vi "Read Username.vi"(8 "error in (no error)":errorcluster, 11 "Player in":refnum<class "Player.lvclass">) -> (0 "error out":errorcluster, 2 "Username":string, 3 "Player out":refnum<class "Player.lvclass">)   [LabVIEW 2019, in "Player.lvclass"]
uses:
  Player.lvclass
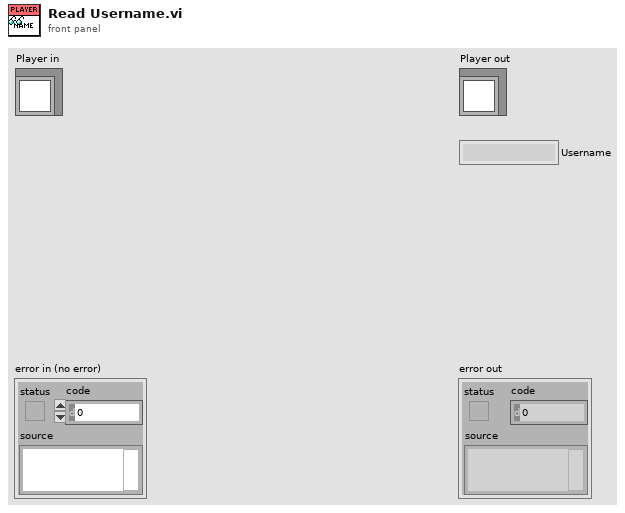
[diagram p1: front panel]
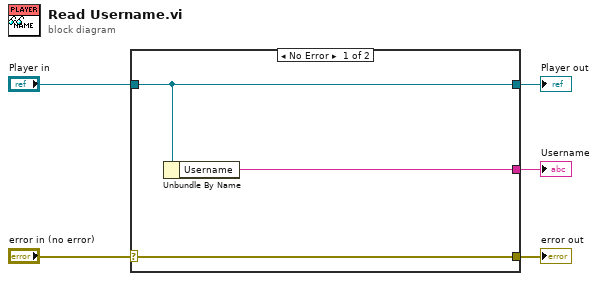
[diagram p0: block diagram]
diagram:
  n1 = case shown="No Error" "error in (no error)" {
    selector: "error in (no error)" -> [w8 w9]
    tunnel: [w8 w9] -> w4
    tunnel: [w7 w10] -> w2
    tunnel: "Player in" -> [w7 w10]
    tunnel: [w6 _] -> w1
    frame No Error {
      n2 = Unbundle By Name(w7) -> ("Username"=w6:string)
    }
    frame Error {
    }
  }
  "error out" <- w4
  "Player out" <- w2
  "Username" <- w1
